vi "Configure Front Panel State.vi"(8 "error in (no error)":errorcluster, 10 "Front Panel State":T1=enum."Standard", 11 "Actor API in":refnum<class "Actor API.lvclass">) -> (0 "error out":errorcluster)   [LabVIEW 2015, in "Actor API.lvclass"]
uses:
  Actor API.lvclass
  Actor/Front Panel State.ctl
  Messaging/Message/Message.lvclass/Message.ctl
  Messaging/Message/Message.lvclass
  Actor/Actor.lvclass
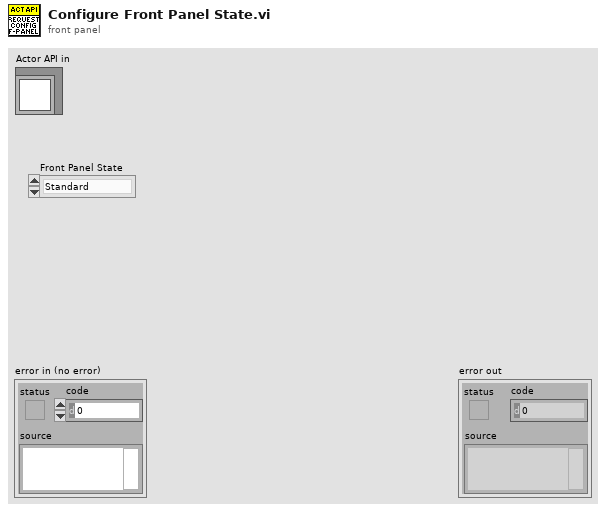
[diagram p1: front panel]
types:
  T1 = typedef "Actor.lvclass/Front Panel State.ctl" = enum32{"Invalid", "Standard", "Closed", "Hidden", "Minimized", "Maximized"}
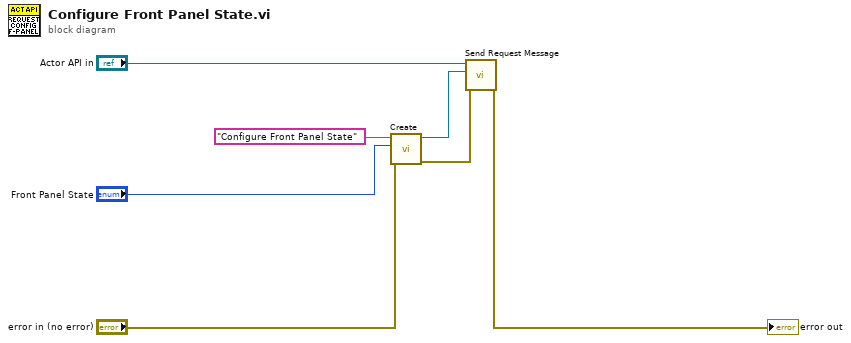
[diagram p0: block diagram]
diagram:
  n1 = call "Create.vi"("error in (no error)"="error in (no error)", "Data"="Front Panel State", "Name"="Configure Front Panel State" ("format string")) -> ("error out"=w1:errorcluster, "Message out"=w2:refnum<class "Message.lvclass">)  [unwired: 7 in]
  n2 = call-dynamic "Send Request Message.vi"("error in (no error)"=w1, "Message"=w2, "Actor API in"="Actor API in") -> ("error out"=→"error out":errorcluster)  [unwired: 8 in]
